vi "NAI5330A.vi"(8 "error in":errorcluster) -> (0 "error out":errorcluster)   [LabVIEW 2020]
uses:
  SubVIs/NAI5330A_TypeDefs.llb/NAI5330A_Button_Internal_External.ctl
  SubVIs/NAI5330A_TypeDefs.llb/NAI5330A_Button_SynRSL.ctl
  SubVIs/NAI5330A_TypeDefs.llb/NAI5330A_Button_Phase.ctl
  SubVIs/NAI5330A_TypeDefs.llb/NAI5330A_Button_VLL.ctl
  SubVIs/NAI5330A_TypeDefs.llb/NAI5330A_Button_Angle.ctl
  SubVIs/NAI5330A_TypeDefs.llb/NAI5330A_Button_FrontRear.ctl
  SubVIs/NAI5330A_TypeDefs.llb/NAI5330A_Button_Mode_Parameter.ctl
  SubVIs/NAI5330A_TypeDefs.llb/NAI5330A_ModeSelector.ctl
  <vilib>/Utility/miscctls.llb/LVPointTypeDef.ctl
  LabVIEW 2020 Toolkits/toolkits_lv2020_32bit/Synchronization.llb/SynchRefs_SetGet.ctl
  SubVIs/NAI5330A_TypeDefs.llb/NAI5330A_Command.ctl
  LabVIEW 2020 Toolkits/VI Server Toolkit/VI Server Libraries/VI Server_GetControl.llb/VI Server_STR_Get.vi
  LabVIEW 2020 Toolkits/VI Server Toolkit/VI Server Toolkit LV2013.lvlib
panel:
  in  "Ch1.FRT/BCK":T1
  in  "UDP.Setup":bool
  in  "Help":bool
  in  "FP.Hide":bool caption="FrontPanel.Hide"
  in  "EXIT":bool
  in  "Tab.Main":T2(tab)
  out "System.Message":string
  in  "Tab.Setup":bool caption="Tab.Ch1.Help"
  in  "Ch1.V.Ref":bool caption="VRef"
  out "Ch1.DynamicMode.Rate":dbl caption="Rate:" format="%0.4f"
  in  "Ch1.Angle.Increment":T3 caption="Angle"
  out "Ch1.DynamicMode.Frequency":dbl caption="Freq:" format="%0.1f"
  out "Ch1.DynamicMode.Amplitude":dbl caption="Amp:" format="%0.4f"
  in  "Ch1.Dynamic.Mode.Parameter":T4
  in  "Ch1.Dynamic.Mode.Selector":T5
  in  "Ch1.Phase.Set.Value":dbl format="%0.1f"
  in  "Ch1.Output":bool caption="ON"
  in  "Ch1.SYN/RSL":T6 caption="RSL"
  in  "Ch1.Internal/External.Ref":T7 caption="FRT"
  in  "Ch1.Angle":dbl caption="Degree" format="%0.3f"
  in  "Ch1.Phase":T8 caption="Phase"
  in  "Ch1.VLL":T9 caption="VLL"
  in  "Ch1.VLL.Set.Value":dbl format="%0.1f"
  in  "Ch1.Ref.Voltage":dbl format="%0.1f"
  in  "Ch1.Mode.Fixed.Ratiometric":bool caption="Mode"
  out "Ch1.Meas.Current":dbl caption="Meas Curr:" format="%0.0f mA"
  out "Ch1.Frequency":dbl caption="Freq:" format="%0.2f Hz"
  out "Ch1.Line-to-Line.Voltage.Measured":dbl caption="Meas VLL:" format="%0.1f V"
  out "Ch1.Ref.Voltage.Measured":dbl caption="Meas VRef:" format="%0.1f V"
  in  "Ch1.Delta":dbl caption="Delta" format="%0.3f"
  in  "Tab.Ch1.Ch1":bool
  in  "Tab.Ch1.Help":bool
  in  "DynamicUpdate.Disable":bool caption="Dynamic Update"
  in  "UpdateTime.Degrees":u32=5 caption="Degrees" min=5 max=20000 format="%d msec"
  in  "UpdateTime.Ref.Parameters":u32=5 caption="Ref. Data" min=5 max=20000 format="%d msec"
  in  "MonitorCommandExecutionStatus":bool caption="Monitor Command Execution Status"
  in  "TCP/IP.Command.Send":bool
  out "TCP/IP.InstrumentResponce":string caption="Instrument Responce"
  in  "TCP/IP.Command":string="*IDN?" caption="Command"
  in  "TCP/IP.Instrument.ID":string="NORTH ATLANTIC,5330A-10" caption="TCP/IP: Instrument ID"
  in  "TCP/IP.Port":u16=23 caption="TCP/IP: Port"
  in  "TCP/IP.Address":string="192.168.4.5" caption="TCP/IP: Address"
  in  "Setup.DONE":bool caption="Ratio.DONE"
  out "UDP.Responce.String":string caption="UDP: Responce String"
  in  "UDP.Responce.String.Monitor":bool
  in  "UDP.Test.String2.Send":bool
  in  "UDP.Test.String2":string caption="UDP: Test String 2"
  in  "UDP.IP.Address":string caption="UDP: IP Address"
  in  "UDP.LocalPort.Write":u16 caption="UDP: Local Port.Write"
  in  "UDP.Port.RT":u16 caption="UDP: Port.RT"
  in  "UDP.Port.BC":u16 caption="UDP: Port.BC"
  in  "UDP.Test.String1":string caption="UDP: Test String 1"
  in  "UDP.Test.String1.Send":bool
  in  "Setup.AdobeAcrobat.Path":path caption="Adobe Acrobat Path"
  in  "AveAnglesReadings.DONE":bool
  in  "Ratio.Value":u8=1 caption="Ratio                              : 1" min=1
  in  "Ratio.Mode":bool
  in  "Ratio.DONE":bool
  in  "Inst.Communication..DONE":bool
  in  "RotationalMode.StartStop":bool caption="Stop/Start"
  out "RotationalMode.Rate.Indicator":bool caption="Rot Rate"
  in  "RotationalMode.Mode":bool caption="Mode"
  in  "RotationalMode.StopAngle":dbl caption="Degree" format="%0.3f"
  out "RotationalMode.StopAngle.Indicator":bool caption="Angle"
  in  "RotationalMode.Angle":dbl caption="Degree" format="%0.3f"
  out "RotationalMode.Angle.Indicator":bool caption="Angle"
  in  "RotationalMode.Rate":dbl caption="Ch1.VLL.Set.Value" format="%0.4f d/s"
  in  "RotationalMode.DONE":bool caption="Ratio.DONE"
  in  "SineWaveMode.DONE":bool caption="Ratio.DONE"
  out "SineWaveMode.Amplitude.Indicator":bool caption="Angle"
  in  "SineWaveMode.Amplitude":dbl caption="Ch1.VLL.Set.Value" format="%0.3f"
  out "SineWaveMode.Frequency.Indicator":bool caption="Angle"
  in  "SineWaveMode.Frequency":dbl caption="Ch1.VLL.Set.Value" format="%0.4f"
  in  "SineWaveMode.StartStop":bool caption="Stop/Start"
  in  "RampWaveMode.DONE":bool caption="Ratio.DONE"
  out "RampWaveMode.Amplitude.Indicator":bool caption="Angle"
  in  "RampWaveMode.Amplitude":dbl caption="Ch1.VLL.Set.Value" format="%0.3f"
  out "RampWaveMode.Frequency.Indicator":bool caption="Angle"
  in  "RampWaveMode.Frequency":dbl caption="Ch1.VLL.Set.Value" format="%0.4f"
  in  "RampWaveMode.StartStop":bool caption="Stop/Start"
  in  "SquareWaveMode.DONE":bool caption="Ratio.DONE"
  out "SquareWaveMode.Amplitude.Indicator":bool caption="Angle"
  in  "SquareWaveMode.Amplitude":dbl caption="Ch1.VLL.Set.Value" format="%0.3f"
  out "SquareWaveMode.Frequency.Indicator":bool caption="Angle"
  in  "SquareWaveMode.Frequency":dbl caption="Ch1.VLL.Set.Value" format="%0.4f"
  in  "SquareWaveMode.StartStop":bool caption="Stop/Start"
  in  "TriangleWaveMode.DONE":bool caption="Ratio.DONE"
  out "TriangleWaveMode.Amplitude.Indicator":bool caption="Angle"
  in  "TriangleWaveMode.Amplitude":dbl caption="Ch1.VLL.Set.Value" format="%0.3f"
  out "TriangleWaveMode.Frequency.Indicator":bool caption="Angle"
  in  "TriangleWaveMode.Frequency":dbl caption="Ch1.VLL.Set.Value" format="%0.4f"
  in  "TriangleWaveMode.StartStop":bool caption="Stop/Start"
  # "Mode:"
  # "Update Time"
  # "Ratio"
  # "Rotation Mode Parameters"
  # "Sine Wave Mode Parameters"
  # "Ramp Wave Mode Parameters"
  # "Square Wave Mode Parameters"
  # "Triangle Wave Mode Parameters"
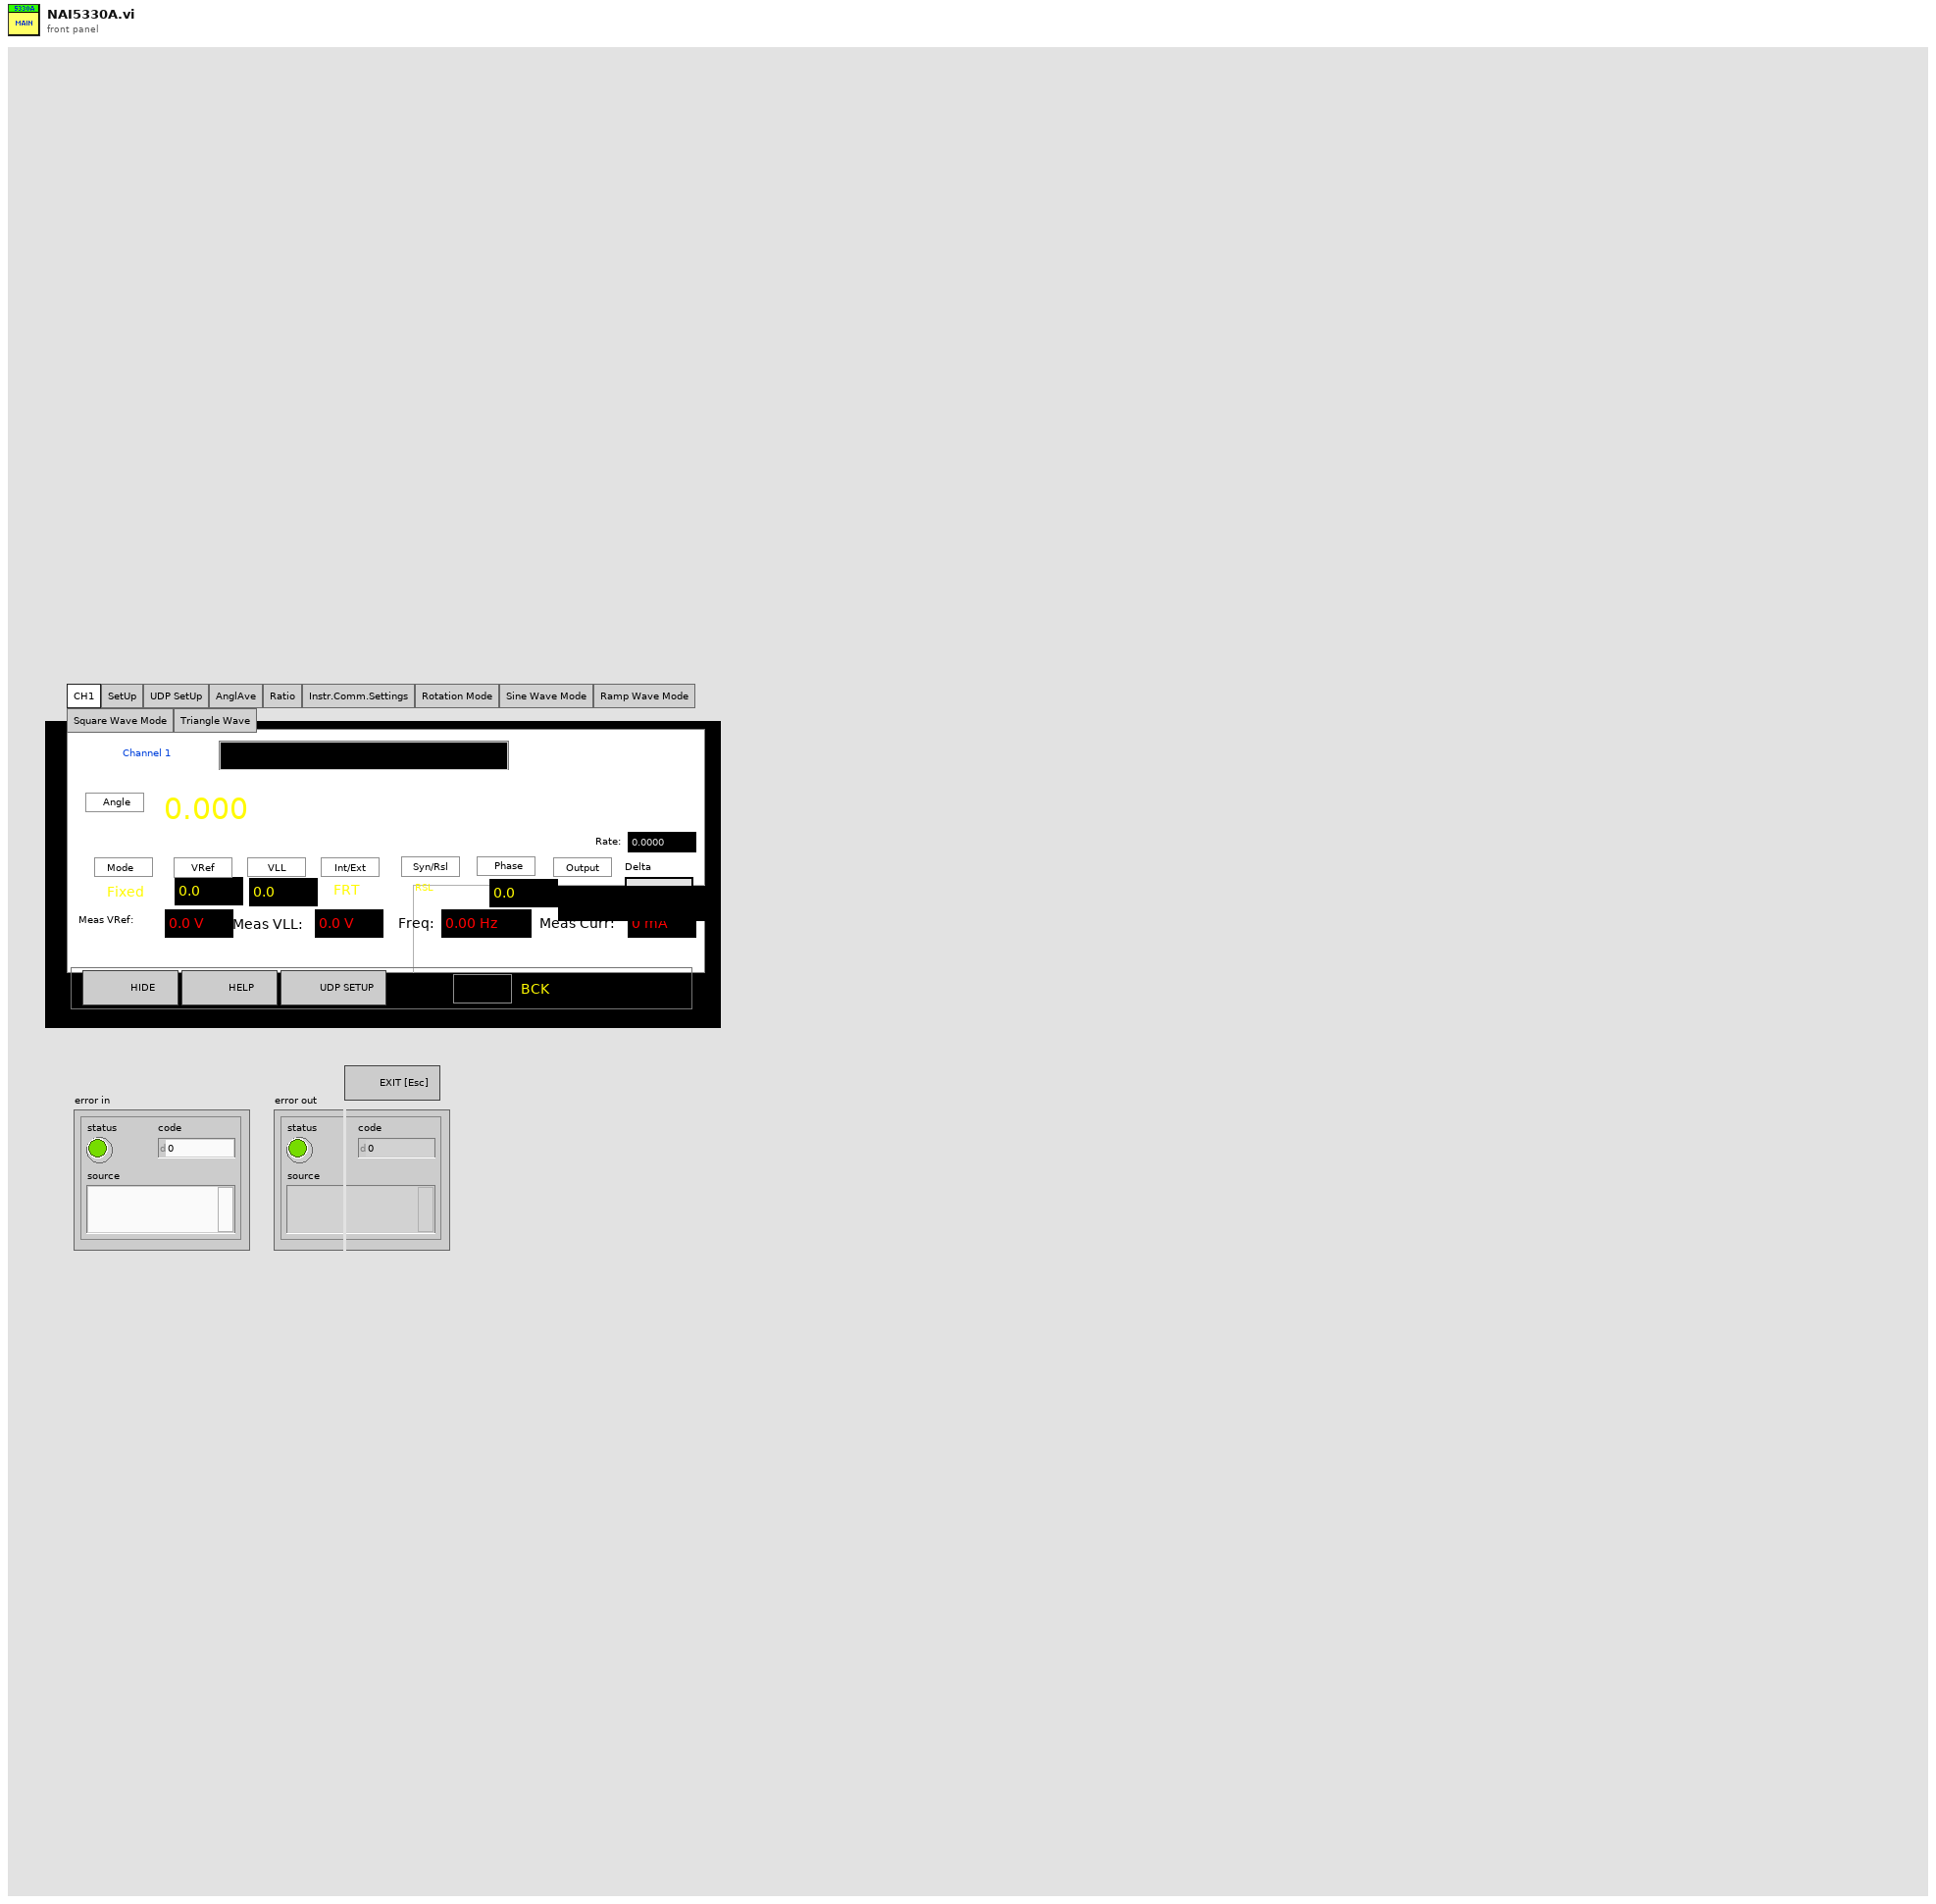
[diagram p1: front panel]
types:
  T1 = typedef "NAI5330A_Button_FrontRear.ctl" = bool
  T2 = enum32{"CH1", "SetUp", "UDP SetUp", "AnglAve", "Ratio", "Instr.Comm.Settings", "Rotation Mode", "Sine Wave Mode", "Ramp Wave Mode", "Square Wave Mode", "Triangle Wave"}
  T3 = typedef "NAI5330A_Button_Angle.ctl" = bool
  T4 = typedef "NAI5330A_Button_Mode_Parameter.ctl" = bool
  T5 = typedef "NAI5330A_ModeSelector.ctl" = u16
  T6 = typedef "NAI5330A_Button_SynRSL.ctl" = bool
  T7 = typedef "NAI5330A_Button_Internal_External.ctl" = bool
  T8 = typedef "NAI5330A_Button_Phase.ctl" = bool
  T9 = typedef "NAI5330A_Button_VLL.ctl" = bool
  T10 = typedef "LVPointTypeDef.ctl" = cluster{"Horizontal":i16, "Vertical":i16}
  T11 = typedef "VI Server_RefsCluster.ctl" = cluster{"Labels":string[], "Refs":refnum<vi>[], "VI Ref":refnum<vi>}
  T12 = typedef "SynchRefs_SetGet.ctl" = enum16{"Set", "Get"}
  T13 = typedef "NAI5330A_Command.ctl" = enum16{"", "*IDN?", "Reference Generator Voltage", "Reference Generator Frequency", "Reference Generator Output State", "Reference Generator Overcurrent State", "Reference Generator Overcurrent State RST ", "Angle Difference", "Angle", "Angle Query", "Reference Voltage", "Angle Ch1-2", "Angle Averaging ON/OFF", "Ch1.Angle Averaged", "Ch2.Angle Averaged", "Angle.AverageRate", "Ch1.Velocity", "Ch2.Velocity", "Line-to-Line Voltage", "Line-to-Line Voltage_Query", "Ch1.ReferenceVoltage", "Ch2.ReferenceVoltage", "Ch1.ReferenceFrequency", "Ch2.ReferenceFrequency", "LOCAL/REMOTE", "ANG_LIMIT.ON|OFF", "ANG_LIMIT.CMP.ABS|ERR", "Ratio", "AngleDisplay.Format", "Angles.Resolution", "Reference Mode", "Channel.Ref.Voltage", "Reference Source", "Signal Mode", "Phase Offset", "Channel Output", "Remote Sense", "Channel 1 Output Connector", "Dynamic Motion Mode", "Dynamic Change?", "Rotation Rate", "Stop Angle", "Dynamic Motion Start/Stop", "Dynamic Motion Amp", "Dynamic Motion Freq", "Ch1.Ref.Voltage.Measured", "Ch1.Line-to-Line.Voltage.Measured", "Ch1.Frequency", "Ch1.Meas.Current"}
  T14 = typedef "Semaphore RefNum" = refnum<k1>
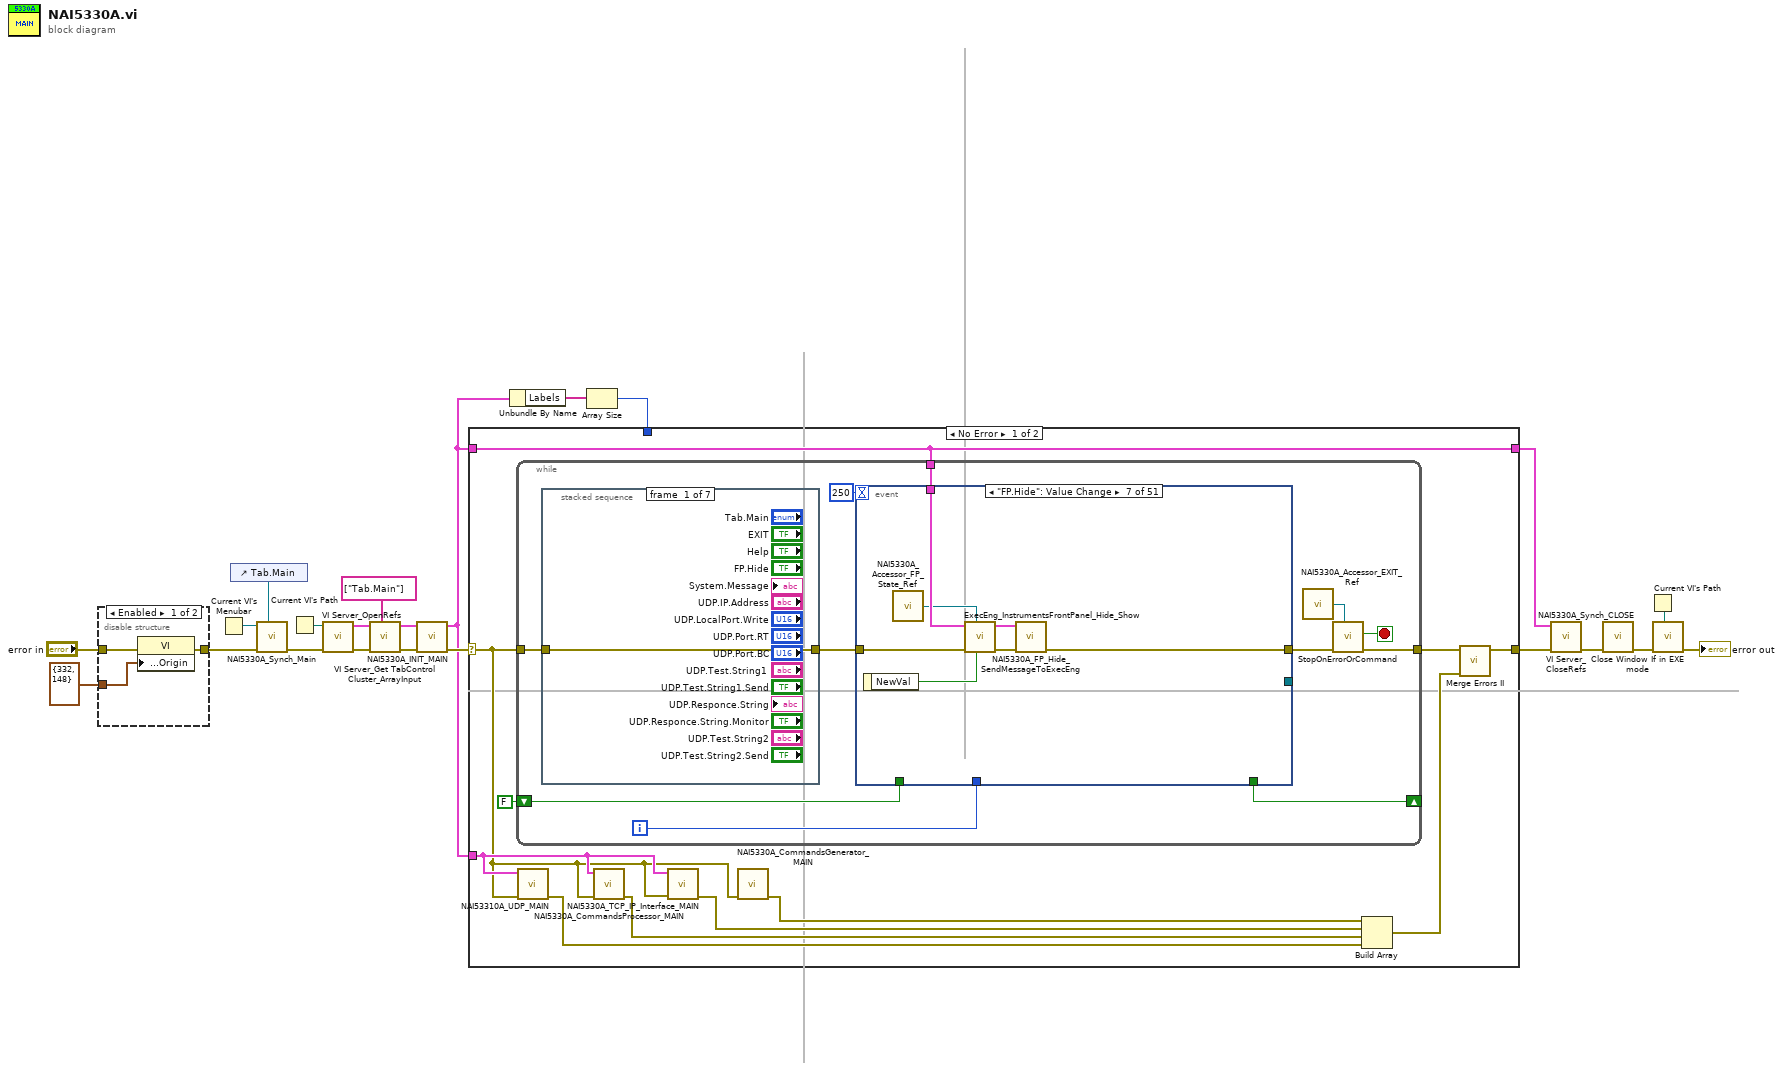
[diagram p0: block diagram]
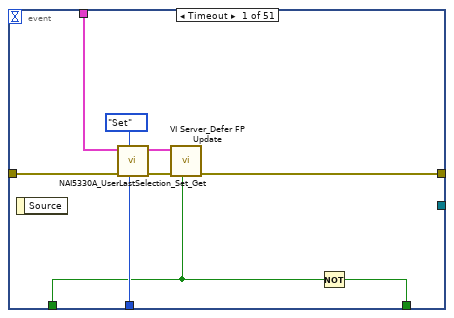
[diagram p3: hidden frame]
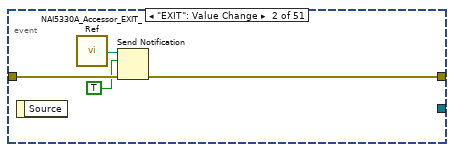
[diagram p4: hidden frame]
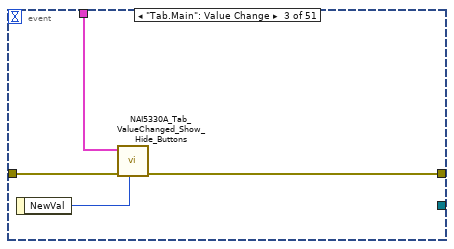
[diagram p5: hidden frame]
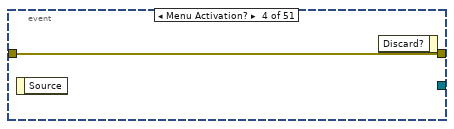
[diagram p6: hidden frame]
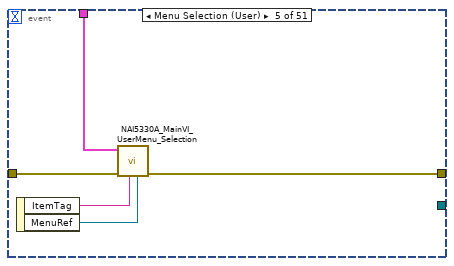
[diagram p7: hidden frame]
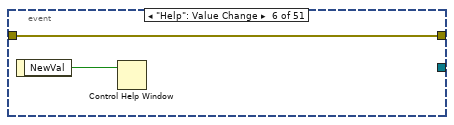
[diagram p8: hidden frame]
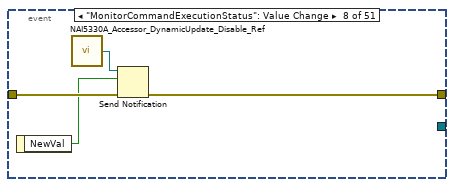
[diagram p9: hidden frame]
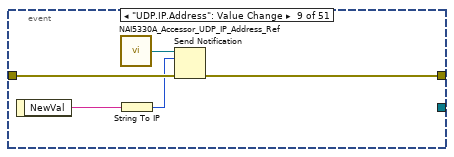
[diagram p10: hidden frame]
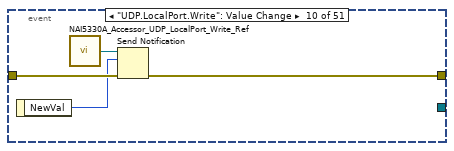
[diagram p11: hidden frame]
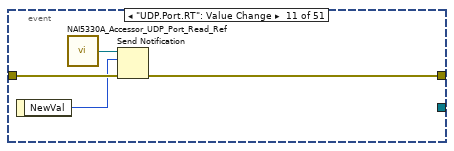
[diagram p12: hidden frame]
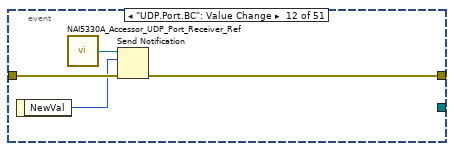
[diagram p13: hidden frame]
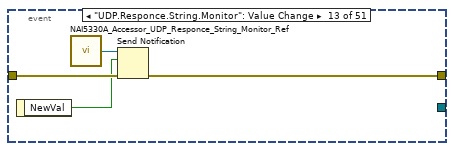
[diagram p14: hidden frame]
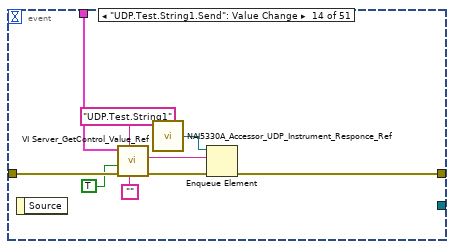
[diagram p15: hidden frame]
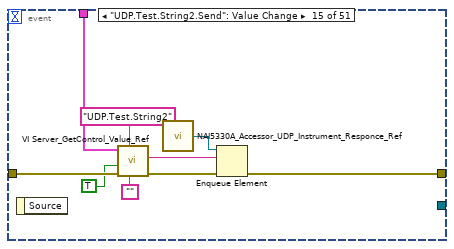
[diagram p16: hidden frame]
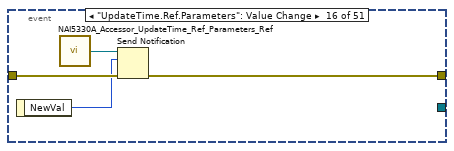
[diagram p17: hidden frame]
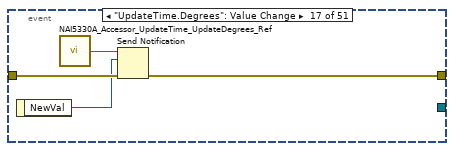
[diagram p18: hidden frame]
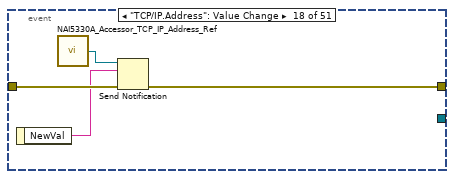
[diagram p19: hidden frame]
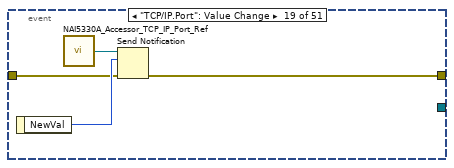
[diagram p20: hidden frame]
diagram:
  n1 = disable-structure shown="Enabled" {
    disable-tunnel: T10 {"Horizontal"=332, "Vertical"=148} ("Front Panel Window:Origin") -> [w25 _]
    disable-tunnel: "error in" -> [w24 w26]
    disable-tunnel: [w23 w26] -> w9
    frame Enabled {
      n2 = property class="VI"(error in=w24, "Front Panel Window:Origin"=w25) -> (error out=w23:errorcluster)  [unwired: 1 in, 1 out]
    }
    frame Disabled {
    }
  }
  n3 = Current VI's Menubar() -> (w4:refnum<k9>)
  n4 = control-ref of="Tab.Main"() -> (w5:refnum<vi>)
  n5 = call "NAI5330A_Synch_Main.vi"("Tab.Main"=w5, "error in"=w9, "menu reference"=w4) -> ("error out"=w12:errorcluster)  [unwired: 8 in]
  n6 = Current VI's Path() -> (path=w19:path)
  n7 = call "VI Server_OpenRefs.vi"("error in"=w12, "VI Path"=w19) -> ("error out"=w22:errorcluster, "VI Server.RefsCluster"=w21:T11)  [unwired: 8 in]
  n8 = call "VI Server_Get TabControl Cluster_ArrayInput.vi"("TabControl Labels[]"=string[] ["Tab.Main"], "error in"=w22, "VI Server Cluster"=w21) -> ("error out"=w14:errorcluster, "VI Server Cluster.OUT"=w13:T11)  [unwired: 7 in]
  n9 = call "NAI5330A_INIT_MAIN.vi"("error in (no error)"=w14, "VI Server Cluster"=w13) -> ("error out"=w15:errorcluster, "VI Server Cluster DUP"=w8:T11)  [unwired: 8 in]
  n10 = Unbundle By Name(w8) -> ("Labels"=w7:string[])
  n11 = Array Size(array=w7) -> (size(s)=w6:i32)
  n12 = case shown="No Error" w15 {
    selector: w15 -> [w29 w281]
    tunnel: [w36 w281] -> w18
    tunnel: w8 -> [w31 _]
    tunnel: w8 -> [w33 w280]
    tunnel: [w33 w280] -> w16
    tunnel: w6 -> [_ _]
    frame No Error {
      n13 = while {
        tunnel: w29 -> [w48]
        tunnel: [w45] -> w37
        tunnel: w33 -> [w41]
        shift-right: [w38] -> _
        shift-left: FALSE -> [w39]
        i -> [w40]
        stop <- w43 stop-if-true
        n14 = stacked-sequence {
          tunnel: w48 -> [w279 _ _ _ _ _ _]
          tunnel: [w279 _ _ _ _ _ _] -> w46
          frame #0 {
          }
          frame #1 {
          }
          frame #2 {
          }
          frame #3 {
          }
          frame #4 {
          }
          frame #5 {
          }
          frame #6 {
          }
        }
        n15 = event shown="[6] \"FP.Hide\": Value Change" {
          selector: _ -> [_ _ _ _ _ _ _ _ _ _ _ _ _ _ _ _ _ _ _ _ _ _ _ _ _ _ _ _ _ _ _ _ _ _ _ _ _ _ _ _ _ _ _ _ _ _ _ _ _ _ _]
          dyn-events: _ -> [_ _ _ _ _ _ _ _ _ _ _ _ _ _ _ _ _ _ _ _ _ _ _ _ _ _ _ _ _ _ _ _ _ _ _ _ _ _ _ _ _ _ _ _ _ _ _ _ _ _ _]
          timeout: 250 -> [_ _ _ _ _ _ _ _ _ _ _ _ _ _ _ _ _ _ _ _ _ _ _ _ _ _ _ _ _ _ _ _ _ _ _ _ _ _ _ _ _ _ _ _ _ _ _ _ _ _ _]
          tunnel: w46 -> [w57 w61 w65 w66 w71 w73 w80 w83 w89 w93 w97 w101 w105 w114 w123 w127 w131 w135 w138 w151 w154 w160 w164 w169 w173 w177 w180 w182 w187 w191 w194 w202 w210 w214 w218 w222 w226 w230 w234 w238 w240 w242 w247 w251 w254 w257 w260 w263 w266 w270 w273]
          tunnel: [w52 w59 w64 w66 w69 w73 w74 w82 w88 w92 w96 w100 w102 w113 w121 w126 w130 w134 w137 w140 w156 w157 w165 w170 w171 w175 w178 w183 w184 w190 w193 w203 w207 w212 w216 w220 w225 w229 w232 w237 w239 w243 w245 w250 w253 w256 w259 w262 w265 w269 w276] -> w44
          tunnel: w41 -> [w56 _ w63 _ w70 _ w78 _ _ _ _ _ _ w112 w120 _ _ _ _ w150 w153 w159 _ _ w172 w176 w179 w181 w186 w189 w192 _ w209 w213 w217 w221 w224 w228 w233 _ _ w241 w246 _ _ _ _ _ _ _ _]
          tunnel: w40 -> [w54 _ _ _ _ _ _ _ _ _ _ _ _ _ _ _ _ _ _ _ _ _ _ _ _ _ _ _ _ _ _ _ _ _ _ _ _ _ _ _ _ _ _ _ _ _ _ _ _ _ _]
          tunnel: [_ _ _ _ _ _ _ _ _ _ _ _ _ _ _ _ _ _ _ _ _ _ _ _ _ w174 _ _ _ _ _ _ _ _ _ _ _ _ _ _ _ _ _ _ _ _ _ _ _ _ _] -> _
          tunnel: w39 -> [w49 _ _ _ _ _ _ _ _ _ _ _ _ _ _ _ _ _ _ _ _ _ _ _ _ _ _ _ _ _ _ _ _ _ _ _ _ _ _ _ _ _ _ _ _ _ _ _ _ _ _]
          tunnel: [w50 _ _ _ _ _ _ _ _ _ _ _ _ _ _ _ _ _ _ _ _ _ _ _ _ _ _ _ _ _ _ _ _ _ _ _ _ _ _ _ _ _ _ _ _ _ _ _ _ _ _] -> w38
          event Timeout {
            n16 = event-data() -> ()  [unwired: 1 in, 1 out]
            n17 = call "NAI5330A_UserLastSelection_Set_Get.vi"("LoopCounter"=w54, "SynchRefs.Set/Get"=SynchRefs_SetGet."Set", "error in"=w57, "VI Server.RefsCluster"=w56) -> ("error out"=w53:errorcluster, "VI Server.RefsCluster.DUP"=w51:T11)  [unwired: 6 in]
            n18 = call "VI Server_Defer FP Update.vi"("Defer Panel Updates? (F)"=w49, "error in"=w53, "VI Server Cluster"=w51) -> ("error out"=w52:errorcluster)  [unwired: 7 in, 1 out]
            n19 = Not(x=w49) -> (.not. x?=w50:bool)
          }
          event "EXIT": Value Change {
            n20 = event-data() -> ()  [unwired: 1 in, 1 out]
            n21 = call "NAI5330A_Accessor_EXIT_Ref.vi"() -> ("EXIT"=w60:refnum<notifier>)  [unwired: 6 in]
            n22 = Send Notification(notification=TRUE, notifier=w60, error in (no error)=w61) -> (error out=w59:errorcluster)  [unwired: 1 out]
          }
          event "Tab.Main": Value Change {
            n23 = event-data() -> ("NewVal"=w62:T2)  [unwired: 1 in]
            n24 = call "NAI5330A_Tab_ValueChanged_Show_Hide_Buttons.vi"("Tab.Main"=w62, "error in (no error)"=w65, "VI Server Cluster"=w63) -> ("error out"=w64:errorcluster)  [unwired: 8 in]
          }
          event Menu Activation? {
            n25 = event-data() -> ()  [unwired: 1 in, 1 out]
            n26 = event-data() -> ()  [unwired: 2 in, 1 out]
          }
          event Menu Selection (User) {
            n27 = event-data() -> ("ItemTag"=w68:string, "MenuRef"=w67:refnum<k9>)  [unwired: 1 in]
            n28 = call "NAI5330A_MainVI_UserMenu_Selection.vi"("MenuRef"=w67, "Menu.ItemTag"=w68, "error in"=w71, "VI Server.RefsCluster"=w70) -> ("error out"=w69:errorcluster)  [unwired: 6 in, 1 out]
          }
          event "Help": Value Change {
            n29 = event-data() -> ("NewVal"=w72:bool)  [unwired: 1 in]
            n30 = Control Help Window(1:w72) -> ()  [unwired: 1 in]
          }
          event "FP.Hide": Value Change {
            n31 = event-data() -> ("NewVal"=w79:bool)  [unwired: 1 in]
            n32 = call "NAI5330A_Accessor_FP_State_Ref.vi"() -> ("FP.State"=w77:refnum<notifier>)  [unwired: 6 in]
            n33 = call "ExecEng_InstrumentsFrontPanel_Hide_Show.vi"("FP.Hide/Show"=w79, "FP.State"=w77, "error in (no error)"=w80, "VI Server Cluster"=w78) -> ("error out"=w76:errorcluster, "VI Server Cluster DUP"=w75:T11)  [unwired: 6 in]
            n34 = call "NAI5330A_FP_Hide_SendMessageToExecEng.vi"("error in (no error)"=w76, "VI Server Cluster"=w75) -> ("error out"=w74:errorcluster)  [unwired: 8 in, 1 out]
          }
          event "MonitorCommandExecutionStatus": Value Change {
            n35 = event-data() -> ("NewVal"=w81:bool)  [unwired: 1 in]
            n36 = call "NAI5330A_Accessor_DynamicUpdate_Disable_Ref.vi"() -> ("DynamicUpdate.Disable"=w84:refnum<notifier>)  [unwired: 6 in]
            n37 = Send Notification(notification=w81, notifier=w84, error in (no error)=w83) -> (error out=w82:errorcluster)  [unwired: 1 out]
          }
          event "UDP.IP.Address": Value Change {
            n38 = event-data() -> ("NewVal"=w86:string)  [unwired: 1 in]
            n39 = call "NAI5330A_Accessor_UDP_IP_Address_Ref.vi"() -> ("UDP.IP.Address"=w87:refnum<notifier>)  [unwired: 6 in]
            n40 = String To IP(1:w86) -> (0:w85:u32)
            n41 = Send Notification(notification=w85, notifier=w87, error in (no error)=w89) -> (error out=w88:errorcluster)  [unwired: 1 out]
          }
          event "UDP.LocalPort.Write": Value Change {
            n42 = event-data() -> ("NewVal"=w90:u16)  [unwired: 1 in]
            n43 = call "NAI5330A_Accessor_UDP_LocalPort_Write_Ref.vi"() -> ("UDP.LocalPort.Write"=w91:refnum<notifier>)  [unwired: 6 in]
            n44 = Send Notification(notification=w90, notifier=w91, error in (no error)=w93) -> (error out=w92:errorcluster)  [unwired: 1 out]
          }
          event "UDP.Port.RT": Value Change {
            n45 = event-data() -> ("NewVal"=w95:u16)  [unwired: 1 in]
            n46 = call "NAI5330A_Accessor_UDP_Port_Read_Ref.vi"() -> ("UDP.Port.Read"=w94:refnum<notifier>)  [unwired: 6 in]
            n47 = Send Notification(notification=w95, notifier=w94, error in (no error)=w97) -> (error out=w96:errorcluster)  [unwired: 1 out]
          }
          event "UDP.Port.BC": Value Change {
            n48 = event-data() -> ("NewVal"=w99:u16)  [unwired: 1 in]
            n49 = call "NAI5330A_Accessor_UDP_Port_Receiver_Ref.vi"() -> ("UDP.Port.Receiver"=w98:refnum<notifier>)  [unwired: 6 in]
            n50 = Send Notification(notification=w99, notifier=w98, error in (no error)=w101) -> (error out=w100:errorcluster)  [unwired: 1 out]
          }
          event "UDP.Responce.String.Monitor": Value Change {
            n51 = event-data() -> ("NewVal"=w104:bool)  [unwired: 1 in]
            n52 = call "NAI5330A_Accessor_UDP_Responce_String_Monitor_Ref.vi"() -> ("UDP.ExecEng.Command.String.Monitor"=w103:refnum<notifier>)  [unwired: 6 in]
            n53 = Send Notification(notification=w104, notifier=w103, error in (no error)=w105) -> (error out=w102:errorcluster)  [unwired: 1 out]
          }
          event "UDP.Test.String1.Send": Value Change {
            n54 = event-data() -> ()  [unwired: 1 in, 1 out]
            n55 = call-poly "VI Server_GetControl_Value_Ref.vi"("DataType"="", "Control.Label"="UDP.Test.String1", "error in"=w114, "SingleInstance"=TRUE, "VI Server.RefsCluster"=w112) -> ("error out"=w106:errorcluster, "Value"=w107:string)  [unwired: 3 in, 2 out]
            n56 = call "NAI5330A_Accessor_UDP_Instrument_Responce_Ref.vi"() -> ("UDP.Instrument.Responce.Q"=w108:refnum<queue>)  [unwired: 6 in]
            n57 = Enqueue Element(queue=w108, element=w107, error in (no error)=w106) -> (error out=w113:errorcluster)  [unwired: 1 in, 2 out]
          }
          event "UDP.Test.String2.Send": Value Change {
            n58 = event-data() -> ()  [unwired: 1 in, 1 out]
            n59 = call-poly "VI Server_GetControl_Value_Ref.vi"("DataType"="", "Control.Label"="UDP.Test.String2", "error in"=w123, "SingleInstance"=TRUE, "VI Server.RefsCluster"=w120) -> ("error out"=w122:errorcluster, "Value"=w116:string)  [unwired: 3 in, 2 out]
            n60 = call "NAI5330A_Accessor_UDP_Instrument_Responce_Ref.vi"() -> ("UDP.Instrument.Responce.Q"=w115:refnum<queue>)  [unwired: 6 in]
            n61 = Enqueue Element(queue=w115, element=w116, error in (no error)=w122) -> (error out=w121:errorcluster)  [unwired: 1 in, 2 out]
          }
          event "UpdateTime.Ref.Parameters": Value Change {
            n62 = event-data() -> ("NewVal"=w124:u32)  [unwired: 1 in]
            n63 = call "NAI5330A_Accessor_UpdateTime_Ref_Parameters_Ref.vi"() -> ("UpdateTime.Ref.Parameters"=w125:refnum<notifier>)  [unwired: 6 in]
            n64 = Send Notification(notification=w124, notifier=w125, error in (no error)=w127) -> (error out=w126:errorcluster)  [unwired: 1 out]
          }
          event "UpdateTime.Degrees": Value Change {
            n65 = event-data() -> ("NewVal"=w128:u32)  [unwired: 1 in]
            n66 = call "NAI5330A_Accessor_UpdateTime_UpdateDegrees_Ref.vi"() -> ("UpdateTime.Degrees"=w129:refnum<notifier>)  [unwired: 6 in]
            n67 = Send Notification(notification=w128, notifier=w129, error in (no error)=w131) -> (error out=w130:errorcluster)  [unwired: 1 out]
          }
          event "TCP/IP.Address": Value Change {
            n68 = event-data() -> ("NewVal"=w133:string)  [unwired: 1 in]
            n69 = call "NAI5330A_Accessor_TCP_IP_Address_Ref.vi"() -> ("TCP/IP.Address"=w132:refnum<notifier>)  [unwired: 6 in]
            n70 = Send Notification(notification=w133, notifier=w132, error in (no error)=w135) -> (error out=w134:errorcluster)  [unwired: 1 out]
          }
          event "TCP/IP.Port": Value Change {
            n71 = event-data() -> ("NewVal"=w139:u16)  [unwired: 1 in]
            n72 = call "NAI5330A_Accessor_TCP_IP_Port_Ref.vi"() -> ("TCP/IP.Port"=w136:refnum<notifier>)  [unwired: 6 in]
            n73 = Send Notification(notification=w139, notifier=w136, error in (no error)=w138) -> (error out=w137:errorcluster)  [unwired: 1 out]
          }
          event "TCP/IP.Command.Send": Value Change {
            n74 = event-data() -> ()  [unwired: 1 in, 1 out]
            n75 = call-poly "VI Server_GetControl_Value_Ref.vi"("DataType"="", "Control.Label"="TCP/IP.Command", "error in"=w151, "SingleInstance"=TRUE, "VI Server.RefsCluster"=w150) -> ("error out"=w145:errorcluster, "Value"=w143:string, "VI Server.RefsCluster.DUP"=w141:T11)  [unwired: 3 in, 1 out]
            n76 = Format Into String(format string="%s\r\n", error in=w145, w143) -> (resulting string=w142:string, error out=w144:errorcluster)  [unwired: 1 in]
            n77 = call "NAI5330A_WriteToInstrument.vi"("error in"=w144, "Command"=w142, "VI Server.RefsCluster"=w141) -> ("error out"=w140:errorcluster)  [unwired: 7 in, 1 out]
          }
          event "Tab.Ch1.Help", "UDP.Setup", "Tab.Setup", "Setup.DONE": Value Change {
            n78 = event-data() -> ("CtlRef"=w155:refnum<vi>)  [unwired: 1 in]
            n79 = control-ref of="Tab.Main"() -> (w152:refnum<vi>)
            n80 = call "NAI5330A_TabSwitch.vi"("CtlRef"=w155, "Tab.Main"=w152, "error in"=w154, "VI Server Cluster"=w153) -> ("error out"=w156:errorcluster)  [unwired: 7 in]
          }
          event "Ch1.Angle": Value Change {
            n81 = event-data() -> ("CtlRef"=w158:refnum<vi>)  [unwired: 1 in]
            n82 = call "NAI5330A_AngleSet.vi"("CtlRef"=w158, "error in (no error)"=w160, "VI Server Cluster"=w159) -> ("error out"=w157:errorcluster)  [unwired: 7 in, 1 out]
          }
          event "Ch1.Angle": Mouse Enter {
            n83 = event-data() -> ()  [unwired: 1 in, 1 out]
            n84 = call "NAI5330A_Accessor_UpdateAnglesSemaphore_Ref.vi"() -> ("UpdateAngles.Semaphore"=w163:T14)  [unwired: 6 in]
            n85 = call "Semaphore_Acquire.vi"("error in"=w164, "SemaphoreRef"=w163) -> ("error out"=w162:errorcluster)  [unwired: 8 in, 1 out]
            n86 = call "NAI5330A_Accessor_UpdateRefParams_Semaphore_Ref.vi"() -> ("UpdateRefParams.Semaphore"=w161:T14)  [unwired: 6 in]
            n87 = call "Semaphore_Acquire.vi"("error in"=w162, "SemaphoreRef"=w161) -> ("error out"=w165:errorcluster)  [unwired: 8 in, 1 out]
          }
          event "Ch1.Angle": Mouse Leave {
            n88 = event-data() -> ()  [unwired: 1 in, 1 out]
            n89 = call "NAI5330A_Accessor_UpdateAnglesSemaphore_Ref.vi"() -> ("UpdateAngles.Semaphore"=w168:T14)  [unwired: 6 in]
            n90 = call "Semaphore_Release.vi"("error in"=w169, "SemaphoreRef"=w168) -> ("error out"=w167:errorcluster)  [unwired: 8 in, 1 out]
            n91 = call "NAI5330A_Accessor_UpdateRefParams_Semaphore_Ref.vi"() -> ("UpdateRefParams.Semaphore"=w166:T14)  [unwired: 6 in]
            n92 = call "Semaphore_Release.vi"("error in"=w167, "SemaphoreRef"=w166) -> ("error out"=w170:errorcluster)  [unwired: 8 in, 1 out]
          }
          event Value Change {
            n93 = event-data() -> ()  [unwired: 1 in, 1 out]
            n94 = call "NAI5330A_AngleIncrement.vi"("error in (no error)"=w173, "VI Server Cluster"=w172) -> ("error out"=w171:errorcluster)  [unwired: 8 in, 1 out]
          }
          event "Ch1.Output", "Tab.Ch1.Ch1", "Tab.Ch1.Help", "Ch1.Mode.Fixed.Ratiometric", "FP.Hide", "UDP.Setup", "EXIT", "AveAnglesReadings.DONE", "Ratio.DONE", "Inst.Communication..DONE", "Ratio.Mode": Mouse Enter {
            n95 = event-data() -> ("CtlRef"=w174:refnum<vi>)  [unwired: 1 in]
            n96 = call "VI Server_SetCursor_HAND.vi"("error in"=w177, "VI Server.RefsCluster"=w176) -> ("error out"=w175:errorcluster)  [unwired: 8 in, 1 out]
          }
          event "Ch1.Output", "Tab.Ch1.Ch1", "Tab.Ch1.Help", "Ch1.Mode.Fixed.Ratiometric", "FP.Hide", "UDP.Setup", "EXIT", "AveAnglesReadings.DONE", "Ratio.DONE", "Inst.Communication..DONE", "Ratio.Mode": Mouse Leave {
            n97 = event-data() -> ()  [unwired: 1 in, 1 out]
            n98 = call "VI Server_SetCursor_ARROW.vi"("error in"=w180, "VI Server.RefsCluster"=w179) -> ("error out"=w178:errorcluster)  [unwired: 8 in, 1 out]
          }
          event Value Change {
            n99 = event-data() -> ()  [unwired: 1 in, 1 out]
            n100 = call "NAI5330A_Ch1_ReferenceSourceSelect.vi"("error in (no error)"=w182, "VI Server.RefsCluster"=w181) -> ("error out"=w183:errorcluster)  [unwired: 8 in, 1 out]
          }
          event Value Change {
            # "ON = SYN; OFF =RES"
            n101 = event-data() -> ("CtlRef"=w185:refnum<vi>)  [unwired: 1 in]
            n102 = call "NAI5330A_Synchro_Resolbver_Mode_Select.vi"("CtlRef"=w185, "error in (no error)"=w187, "VI Server Cluster"=w186) -> ("error out"=w184:errorcluster)  [unwired: 7 in, 1 out]
          }
          event "Ch1.Mode.Fixed.Ratiometric": Value Change {
            n103 = event-data() -> ("CtlRef"=w188:refnum<vi>)  [unwired: 1 in]
            n104 = call "NAI5330A_Reference_Mode.vi"("CtlRef"=w188, "error in"=w191, "VI Server.RefsCluster"=w189) -> ("error out"=w190:errorcluster)  [unwired: 7 in, 1 out]
          }
          event "Ratio.Mode": Value Change {
            n105 = event-data() -> ()  [unwired: 1 in, 1 out]
            n106 = call "NAI5330A_Ratio_Mode.vi"("error in"=w194, "VI Server.RefsCluster"=w192) -> ("error out"=w193:errorcluster)  [unwired: 8 in, 1 out]
          }
          event Value Change {
            # "ON = BACK; OFF =FRONT"
            n107 = event-data() -> ("NewVal"=w201:T1)  [unwired: 1 in]
            n108 = call "NAI5330A_Accessor_Command_Value1_Ref.vi"() -> ("Command.Value.1"=w205:refnum<notifier>)  [unwired: 6 in]
            n109 = Select(t="FRONT", s=w201, f="BACK") -> (s? t:f=w204:string)
            n110 = Send Notification(notification=w204, notifier=w205, error in (no error)=w202) -> (error out=w196:errorcluster)  [unwired: 1 out]
            n111 = call "NAI5330A_Accessor_Command_Ref.vi"() -> ("Command"=w198:refnum<queue>)  [unwired: 6 in]
            n112 = Flush Queue(queue=w198, error in (no error)=w196) -> (queue out=w197:refnum<queue>, error out=w195:errorcluster)  [unwired: 1 out]
            n113 = Enqueue Element(queue=w197, element=NAI5330A_Command."Channel 1 Output Connector", error in (no error)=w195) -> (error out=w203:errorcluster)  [unwired: 1 in, 2 out]
          }
          event "Ch1.V.Ref": Value Change {
            n114 = event-data() -> ("CtlRef"=w208:refnum<vi>)  [unwired: 1 in]
            n115 = call "NAI5330A_Message_EnterChannelRef_Voltage.vi"("CtlRef"=w208, "error in"=w210, "VI Server.RefsCluster"=w209) -> ("error out"=w207:errorcluster)  [unwired: 7 in, 1 out]
          }
          event "Ch1.Ref.Voltage": Value Change {
            n116 = event-data() -> ("CtlRef"=w211:refnum<vi>)  [unwired: 1 in]
            n117 = call "NAI5330A_ChannelRef_Voltage.vi"("CtlRef"=w211, "error in"=w214, "VI Server.RefsCluster"=w213) -> ("error out"=w212:errorcluster)  [unwired: 7 in, 1 out]
          }
          event Value Change {
            n118 = event-data() -> ("CtlRef"=w215:refnum<vi>)  [unwired: 1 in]
            n119 = call "NAI5330A_Message_EnterChannel_VLL.vi"("CtlRef"=w215, "error in"=w218, "VI Server.RefsCluster"=w217) -> ("error out"=w216:errorcluster)  [unwired: 7 in, 1 out]
          }
          event "Ch1.VLL.Set.Value": Value Change {
            n120 = event-data() -> ("CtlRef"=w219:refnum<vi>)  [unwired: 1 in]
            n121 = call "NAI5330A_Channel_VLL.vi"("CtlRef"=w219, "error in"=w222, "VI Server.RefsCluster"=w221) -> ("error out"=w220:errorcluster)  [unwired: 7 in, 1 out]
          }
          event Value Change {
            n122 = event-data() -> ("CtlRef"=w223:refnum<vi>)  [unwired: 1 in]
            n123 = call "NAI5330A_Message_Enter_Phase_Offset.vi"("CtlRef"=w223, "error in"=w226, "VI Server.RefsCluster"=w224) -> ("error out"=w225:errorcluster)  [unwired: 7 in, 1 out]
          }
          event "Ch1.Phase.Set.Value": Value Change {
            n124 = event-data() -> ("CtlRef"=w227:refnum<vi>)  [unwired: 1 in]
            n125 = call "NAI5330A_Phase_Offset.vi"("CtlRef"=w227, "error in"=w230, "VI Server.RefsCluster"=w228) -> ("error out"=w229:errorcluster)  [unwired: 7 in, 1 out]
          }
          event "Ch1.Output": Value Change {
            n126 = event-data() -> ("CtlRef"=w231:refnum<vi>)  [unwired: 1 in]
            n127 = call "NAI5330A_Channel_Output.vi"("CtlRef"=w231, "error in"=w234, "VI Server.RefsCluster"=w233) -> ("error out"=w232:errorcluster)  [unwired: 7 in, 1 out]
          }
          event "Ch1.Ref.Voltage.Measured", "Ch1.Line-to-Line.Voltage.Measured", "Ch1.Frequency", "Ch1.Meas.Current": Shortcut Menu Selection (User) {
            n128 = event-data() -> ("CtlRef"=w236:refnum<vi>, "ItemTag"=w235:string)  [unwired: 1 in]
            n129 = call "NAI5330A_UpdateIndicators.vi"("ItemTag"=w235, "Ctl.Ref"=w236, "error in (no error)"=w238) -> ("error out"=w237:errorcluster)  [unwired: 8 in]
          }
          event "AveAnglesReadings.DONE", "Ratio.DONE", "Inst.Communication..DONE": Value Change {
            n130 = event-data() -> ()  [unwired: 1 in, 1 out]
            n131 = call "NAI5330A_AverageAngleReadings_DONE.vi"("error in"=w240) -> ("error out"=w239:errorcluster)  [unwired: 10 in]
          }
          event Value Change {
            n132 = event-data() -> ()  [unwired: 1 in, 1 out]
            n133 = call "NAI5330A_DynamicModeParameter.vi"("error in (no error)"=w242, "VI Server Cluster"=w241) -> ("error out"=w243:errorcluster)  [unwired: 9 in]
          }
          event Value Change {
            n134 = event-data() -> ("CtlRef"=w244:refnum<vi>)  [unwired: 1 in]
            n135 = call "NAI5330A_InternalRef_Dynamic_Motion_Mode.vi"("CtlRef"=w244, "error in (no error)"=w247, "VI Server Cluster"=w246) -> ("error out"=w245:errorcluster)  [unwired: 7 in, 1 out]
          }
          event "DynamicUpdate.Disable": Value Change {
            n136 = event-data() -> ("NewVal"=w249:bool)  [unwired: 1 in]
            n137 = call "NAI5330A_Accessor_DynamicUpdate_Disable_Ref.vi"() -> ("DynamicUpdate.Disable"=w248:refnum<notifier>)  [unwired: 6 in]
            n138 = Send Notification(notification=w249, notifier=w248, error in (no error)=w251) -> (error out=w250:errorcluster)  [unwired: 1 out]
          }
          event "RotationalMode.StopAngle": Value Change {
            n139 = event-data() -> ("NewVal"=w252:dbl)  [unwired: 1 in]
            n140 = call "NAI5330_RotationalMode_StopAngle.vi"("StopAngle"=w252, "error in (no error)"=w254) -> ("error out"=w253:errorcluster)  [unwired: 9 in]
          }
          event "RotationalMode.Mode": Value Change {
            n141 = event-data() -> ("NewVal"=w255:bool)  [unwired: 1 in]
            n142 = call "NAI5330_RotationalMode_StartStop_Continious.vi"("Start/Stop/Cont"=w255, "error in (no error)"=w257) -> ("error out"=w256:errorcluster)  [unwired: 9 in]
          }
          event "RotationalMode.Rate": Value Change {
            n143 = event-data() -> ("NewVal"=w258:dbl)  [unwired: 1 in]
            n144 = call "NAI5330_RotationalMode_Rate.vi"("StopAngle"=w258, "error in (no error)"=w260) -> ("error out"=w259:errorcluster)  [unwired: 9 in]
          }
          event "SineWaveMode.Frequency", "RampWaveMode.Frequency", "SquareWaveMode.Frequency", "TriangleWaveMode.Frequency": Value Change {
            n145 = event-data() -> ("NewVal"=w261:dbl)  [unwired: 1 in]
            n146 = call "NAI5330_DynamicMode_Frequency.vi"("StopAngle"=w261, "error in (no error)"=w263) -> ("error out"=w262:errorcluster)  [unwired: 9 in]
          }
          event "SineWaveMode.Amplitude", "RampWaveMode.Amplitude", "SquareWaveMode.Amplitude", "TriangleWaveMode.Amplitude": Value Change {
            n147 = event-data() -> ("NewVal"=w264:dbl)  [unwired: 1 in]
            n148 = call "NAI5330_DynamicMode_Amplitude.vi"("StopAngle"=w264, "error in (no error)"=w266) -> ("error out"=w265:errorcluster)  [unwired: 9 in]
          }
          event "RotationalMode.StartStop", "SineWaveMode.StartStop", "RampWaveMode.StartStop", "SquareWaveMode.StartStop", "TriangleWaveMode.StartStop": Value Change {
            n149 = event-data() -> ("NewVal"=w268:bool, "CtlRef"=w267:refnum<vi>)  [unwired: 1 in]
            n150 = call "NAI5330_DynamicMode_Start_Stop.vi"("CtlRef"=w267, "Start/Stop"=w268, "error in (no error)"=w270) -> ("error out"=w269:errorcluster)  [unwired: 8 in]
          }
          event "RotationalMode.DONE", "SineWaveMode.DONE", "RampWaveMode.DONE", "SquareWaveMode.DONE", "TriangleWaveMode.DONE": Value Change {
            n151 = event-data() -> ()  [unwired: 1 in, 1 out]
            n152 = call "NAI5330A_Accessor_TabMain_PrevPage_Ref.vi"() -> ("Tab.Main.PrevPage"=w272:refnum<notifier>)  [unwired: 6 in]
            n153 = Get Notifier Status(notifier=w272, error in (no error)=w273) -> (current notification=w271:T2, error out=w274:errorcluster)  [unwired: 3 out]
            n154 = call "NAI5330A_Accessor_Tab_Main_Ref.vi"() -> ("Tab.Main.Ref"=w275:refnum<notifier>)  [unwired: 6 in]
            n155 = Get Notifier Status(notifier=w275, error in (no error)=w274) -> (current notification=w278:refnum<vi>, error out=w277:errorcluster)  [unwired: 3 out]
            n156 = property class="TabCtl (strict)"(reference=w278, error in=w277, "Value"=w271) -> (error out=w276:errorcluster)  [unwired: 1 out]
          }
        }
        n157 = call "NAI5330A_Accessor_EXIT_Ref.vi"() -> ("EXIT"=w42:refnum<notifier>)  [unwired: 6 in]
        n158 = call "StopOnErrorOrCommand.vi"("STOP"=w42, "error in (no error)"=w44) -> ("error out"=w45:errorcluster, "STOP"=w43:bool)  [unwired: 8 in]
      }
      n159 = call "NAI53310A_UDP_MAIN.vi"("error in (no error)"=w29, "VI Server.RefsCluster"=w31) -> ("error out"=w35:errorcluster)  [unwired: 9 in]
      n160 = call "NAI5330A_CommandsProcessor_MAIN.vi"("error in"=w29, "VI Server.RefsCluster"=w31) -> ("error out"=w32:errorcluster)  [unwired: 8 in, 1 out]
      n161 = call "NAI5330A_TCP_IP_Interface_MAIN.vi"("error in"=w29, "VI Server.RefsCluster"=w31) -> ("error out"=w30:errorcluster)  [unwired: 9 in]
      n162 = call "NAI5330A_CommandsGenerator_MAIN.vi"("error in"=w29) -> ("error out"=w28:errorcluster)  [unwired: 10 in]
      n163 = Build Array(w28, w30, w32, w35) -> (w34:errorcluster[])
      n164 = call "Merge Errors II.vi"("error array in"=w34, "error in 1 (no error)"=w37) -> ("error out.DUP"=w36:errorcluster)  [unwired: 4 in, 1 out]
    }
    frame Error {
    }
  }
  n165 = call "VI Server_CloseRefs.vi"("error in"=w18, "VI Server.RefsCluster"=w16) -> ("error out"=w17:errorcluster)  [unwired: 9 in]
  n166 = call "NAI5330A_Synch_CLOSE.vi"("error in"=w17) -> ("error out"=w3:errorcluster)  [unwired: 10 in]
  n167 = Current VI's Path() -> (path=w1:path)
  n168 = call "Close Window If in EXE mode.vi"("TopLevelVI Path"=w1, "error in"=w3) -> ("error out"=→"error out":errorcluster)  [unwired: 9 in]
